vi "Send Configure Trigger.vi"(7 "Message Priority (Normal)":T1=enum."Normal", 8 "error in (no error)":errorcluster, 9 "trigger holdoff (500.0 E-9 s)":dbl[unit]=5e-07 format="%^.2e", 10 "trigger type (Edge)":i32(ring)=1 items=["Edge"=1, "TV"=5, "Runt"=3, "Glitch"=4, "Width"=2, "AC Line"=7, "Immediate"=6], 11 "Message Enqueuer":refnum<class "Message Enqueuer.lvclass">) -> (0 "error out":errorcluster, 3 "Message Enqueuer out":refnum<class "Message Enqueuer.lvclass">)   [LabVIEW 2014, in "CS++Scope.lvlib" / "Configure Trigger Msg.lvclass"]
doc: "Sends the <B>CS++Scope.lvlib:Configure Trigger Msg.lvclass</B> message.\n\n<B>CS++Scope.lvlib:CS++Scope.lvclass:Configure Trigger.vi</B> Description:\n\nThis VI configures the common properties of the trigger subsystem. These properties are the trigger type and holdoff.\nWhen you call IviScope Read Waveform, IviScope Read Waveform Measurement [WM], IviScope Read Min Max Waveform [MmW], or IviScope Initiate Acquisition, the oscilloscope waits for a trigger. You specify the type of trigger for which the oscilloscope waits with the Trigger Type parameter.\nIf the oscilloscope requires multiple waveform acquisitions to build a complete waveform, it waits for the length of time you specify with the Holdoff parameter to elapse since the previous trigger. The oscilloscope then waits for the next trigger. Once the oscilloscope acquires a complete waveform, it returns to the Idle state."
uses:
  Configure Trigger Msg.lvclass
  <vilib>/ActorFramework/Message Enqueuer/Message Enqueuer.lvclass
  <vilib>/ActorFramework/Message Enqueuer/Message Priority.ctl
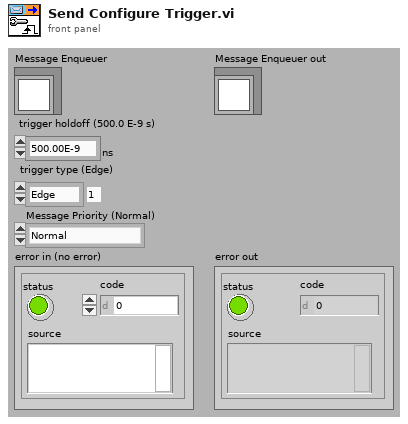
[diagram p1: front panel]
types:
  T1 = typedef "Actor Framework.lvlib/Message Enqueuer.lvclass/Message Priority.ctl" = enum16{"Low", "Normal", "High"}
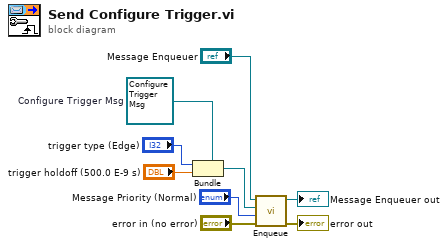
[diagram p0: block diagram]
diagram:
  w3 = refnum<class "Configure Trigger Msg.lvclass"> refnum  # Configure Trigger Msg
  n1 = Bundle(cluster=w3, "trigger type (Edge)", "trigger holdoff (500.0 E-9 s)") -> (w6:refnum<class "Configure Trigger Msg.lvclass">)
  n2 = call <vilib>:"Enqueue.vi"("error in (no error)"="error in (no error)", "Message Priority (Normal)"="Message Priority (Normal)", "Message"=w6, "Message Enqueuer in"="Message Enqueuer") -> ("error out"=→"error out":errorcluster, "Message Enqueuer out"=→"Message Enqueuer out":refnum<class "Message Enqueuer.lvclass">)  [unwired: 6 in]
